vi "Init--Core.vi"(8 "error in (no error)":errorcluster, 11 "EventLogHandle in":refnum<class "EventLogHandle.lvclass">) -> (0 "error out":errorcluster, 3 "EventLogHandle out":refnum<class "EventLogHandle.lvclass">)   [LabVIEW 2024, in "EventLogHandle.lvclass"]
uses:
  EventLogHandle.lvclass
  EventLogHandle.lvclass/EventLogHandle.ctl
  Record/LogRecord.lvclass
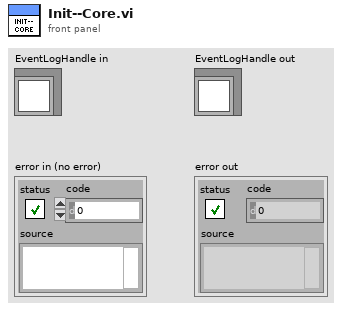
[diagram p1: front panel]
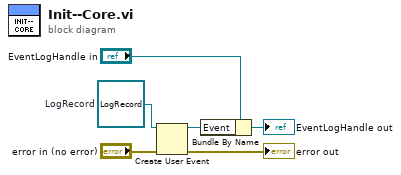
[diagram p0: block diagram]
diagram:
  w6 = refnum<class "LogRecord.lvclass"> refnum  # LogRecord
  n1 = Create User Event(user event datatype=w6, error in="error in (no error)") -> (user event=w4:refnum<user-event>, error out=→"error out":errorcluster)
  n2 = Bundle By Name(cluster="EventLogHandle in", "Event"=w4) -> (→"EventLogHandle out":refnum<class "EventLogHandle.lvclass">)
